vi "CHeckHardware.vi"(3 "Hardware":path) -> (1 "HardwareSpecs":T1)   [LabVIEW 2012]
uses:
  <userlib>/BotSpeak/VIs/SubVIs/BotSpeak.HardwareSpecs.ctl
  <userlib>/BotSpeak/VIs/SubVIs/BotSpeak_Globals.vi
panel:
  out "path":path
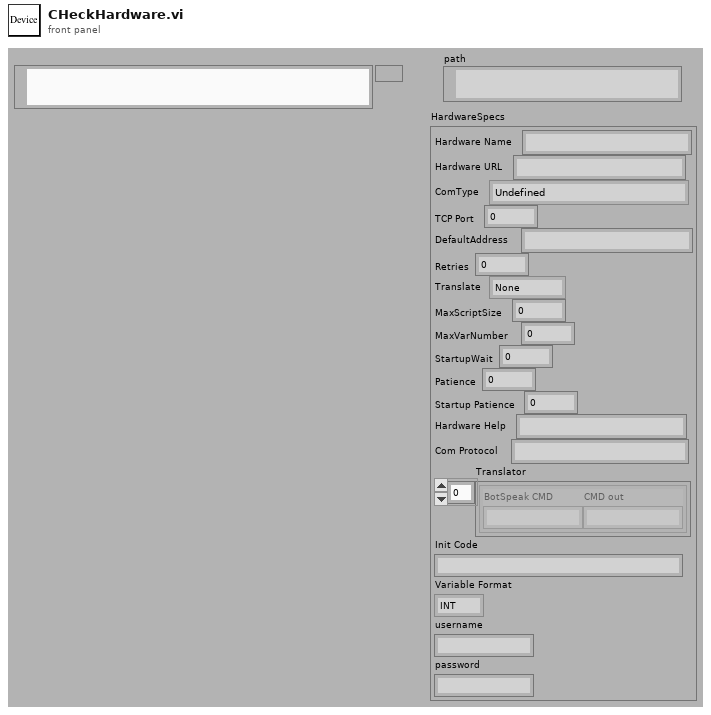
[diagram p1: front panel]
types:
  T1 = typedef "BotSpeak.HardwareSpecs.ctl" = cluster{"Hardware Name":string, "Hardware URL":string, "ComType":enum16{"Undefined", "Serial", "TCPIP", "Console", "EV3"}, "TCP Port":i32, "DefaultAddress":string, "Retries":i32, "Translate":enum16{"None", "Tiny", "URAPI"}, "MaxScriptSize":i32, "MaxVarNumber":i32, "StartupWait":i32, "Patience":i32, "Startup Patience":i32, "Hardware Help":string, "Com Protocol":string, "Translator":cluster{"BotSpeak CMD":string, "CMD out":string}[], "Init Code":string, "Variable Format":enum16{"INT", "FLOAT", "FIXED"}, "username":string, "password":string}
  T2 = typedef "BotSpeak_Control.ctl" = cluster{"Address":string, "Reply EOF":string, "Hardware":string, "Retries":i8, "Timeout":i32, "Open?":bool}
  T3 = cluster{"trimmed string":string, "trimmed string":string}[]
  T4 = cluster{"trimmed string":string, "trimmed string":string}
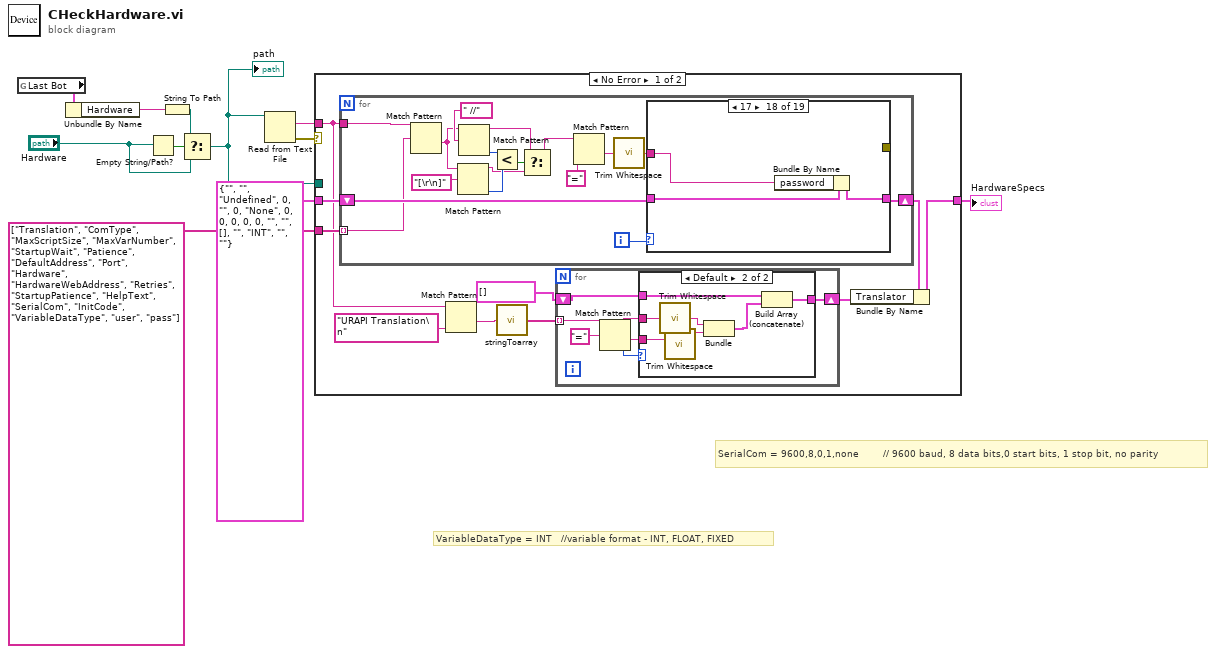
[diagram p0: block diagram]
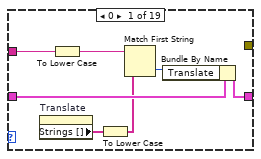
[diagram p3: hidden frame]
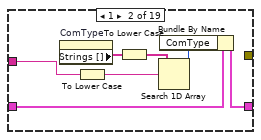
[diagram p4: hidden frame]
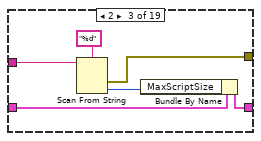
[diagram p5: hidden frame]
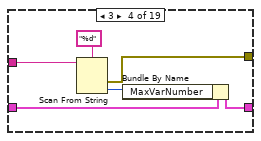
[diagram p6: hidden frame]
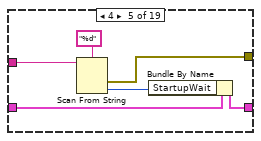
[diagram p7: hidden frame]
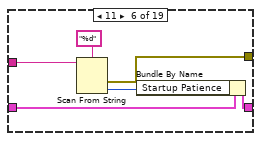
[diagram p8: hidden frame]
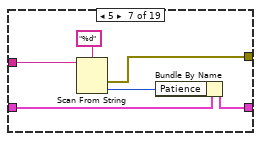
[diagram p9: hidden frame]
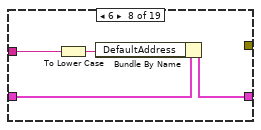
[diagram p10: hidden frame]
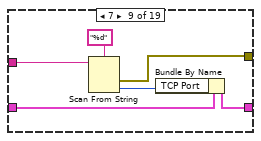
[diagram p11: hidden frame]
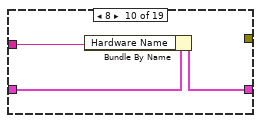
[diagram p12: hidden frame]
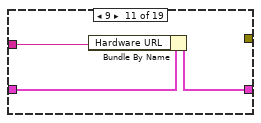
[diagram p13: hidden frame]
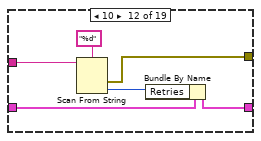
[diagram p14: hidden frame]
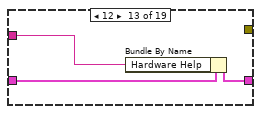
[diagram p15: hidden frame]
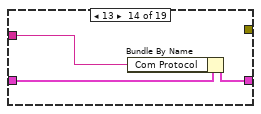
[diagram p16: hidden frame]
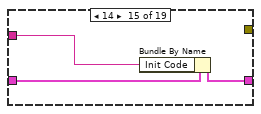
[diagram p17: hidden frame]
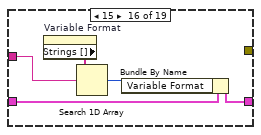
[diagram p18: hidden frame]
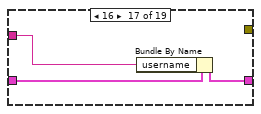
[diagram p19: hidden frame]
diagram:
  # "VariableDataType = INT   //variable format - INT, FLOAT, FIXED"
  # "SerialCom = 9600,8,0,1,none        // 9600 baud, 8 data bits,0 start bits, 1 stop bit, no parity"
  n1 = global read "BotSpeak_Globals.vi" "Last Bot"() -> (w6:T2)
  n2 = Unbundle By Name(w6) -> ("Hardware"=w2:string)
  n3 = Empty String/Path?(string/path="Hardware") -> (empty?=w5:bool)
  n4 = String To Path(string=w2) -> (path=w1:path)
  n5 = Select(t=w1, s=w5, f="Hardware") -> (s? t:f=w3:path)
  "path" <- w3
  n6 = Read from Text File(file (use dialog)=w3) -> (text=w10:string, error out=w11:errorcluster)  [unwired: 3 in, 2 out]
  n7 = case shown="No Error" w11 {
    tunnel: w3 -> [_ w142]
    tunnel: string[] ["Translation", "ComType", "MaxScriptSize", "MaxVarNumber", "StartupWait", "Patience", "DefaultAddress", "Port", "Hardware", "HardwareWebAddress", "Retries", "StartupPatience", "HelpText", "SerialCom", "InitCode", "VariableDataType", "user", "pass"] -> [w21 _]
    tunnel: w10 -> [w19 _]
    tunnel: T1 {"Hardware Name"="", "Hardware URL"="", "ComType"=enum."Undefined", "TCP Port"=0, "DefaultAddress"="", "Retries"=0, "Translate"=enum."None", "MaxScriptSize"=0, "MaxVarNumber"=0, "StartupWait"=0, "Patience"=0, "Startup Patience"=0, "Hardware Help"="", "Com Protocol"="", "Translator"=[], "Init Code"="", "Variable Format"=enum."INT", "username"="", "password"=""} ("HardwareSpecs") -> [w20 w141]
    tunnel: [w14 w141] -> w8
    frame No Error {
      n8 = for {
        tunnel: w21 -> [w42] mode=indexing
        tunnel: w19 -> [w41]
        shift-right: [w49] -> w15
        shift-left: w20 -> [w50]
        i -> [w51]
        n9 = Match Pattern(string=w41, regular expression=w42) -> (after substring=w45:string)  [unwired: 1 in, 3 out]
        n10 = Match Pattern(string=w45, regular expression="[\r\n]") -> (before substring=w39:string, offset past match=w43:i32)  [unwired: 1 in, 2 out]
        n11 = Match Pattern(string=w45, regular expression=" //") -> (before substring=w40:string, offset past match=w44:i32)  [unwired: 1 in, 2 out]
        n12 = Less?(x=w44, y=w43) -> (x < y?=w38:bool)
        n13 = Select(t=w40, s=w38, f=w39) -> (s? t:f=w37:string)
        n14 = Match Pattern(string=w37, regular expression="=") -> (after substring=w52:string)  [unwired: 1 in, 3 out]
        n15 = call <vilib>:"Trim Whitespace.vi"("string"=w52) -> ("trimmed string"=w48:string)  [unwired: 1 in]
        n16 = case shown="17" w51 {
          tunnel: w50 -> [w60 w67 w73 w79 w85 w91 w97 w101 w107 w110 w113 w119 w122 w125 w128 w133 w136 w139 w140]
          tunnel: [w59 w66 w72 w78 w84 w90 w96 w100 w106 w109 w112 w118 w121 w124 w127 w132 w135 w138 w140] -> w49
          tunnel: w48 -> [w58 w65 w71 w77 w83 w89 w95 w99 w105 w108 w111 w117 w120 w123 w126 w130 w134 w137 _]
          tunnel: [_ _ w68 w74 w80 w86 w92 _ w102 _ _ w114 _ _ _ _ _ _ _] -> _
          frame 0 {
            n17 = property on="Translate" class="Enum (strict)"() -> ("Strings []"=w56:string[])  [unwired: 2 in, 2 out]
            n18 = To Lower Case(string=w58) -> (all lower case string=w57:string)
            n19 = To Lower Case(string=w56) -> (all lower case string=w54:string[])
            n20 = Match First String(2:w54, 3:w57) -> (0:w55:i32)  [unwired: 1 out]
            n21 = Bundle By Name(cluster=w60, "Translate"=w55) -> (w59:T1)
          }
          frame 1 {
            n22 = property on="ComType" class="Enum (strict)"() -> ("Strings []"=w62:string[])  [unwired: 2 in, 2 out]
            n23 = To Lower Case(string=w65) -> (all lower case string=w61:string)
            n24 = To Lower Case(string=w62) -> (all lower case string=w63:string[])
            n25 = Search 1D Array(1D array=w63, element=w61) -> (index of element=w64:i32)  [unwired: 1 in]
            n26 = Bundle By Name(cluster=w67, "ComType"=w64) -> (w66:T1)
          }
          frame 2 {
            n27 = Scan From String(format string="%d", input string=w71) -> (error out=w68:errorcluster, output 1=w70:i32)  [unwired: 3 in, 2 out]
            n28 = Bundle By Name(cluster=w73, "MaxScriptSize"=w70) -> (w72:T1)
          }
          frame 3 {
            n29 = Scan From String(format string="%d", input string=w77) -> (error out=w74:errorcluster, output 1=w76:i32)  [unwired: 3 in, 2 out]
            n30 = Bundle By Name(cluster=w79, "MaxVarNumber"=w76) -> (w78:T1)
          }
          frame 4 {
            n31 = Scan From String(format string="%d", input string=w83) -> (error out=w80:errorcluster, output 1=w82:i32)  [unwired: 3 in, 2 out]
            n32 = Bundle By Name(cluster=w85, "StartupWait"=w82) -> (w84:T1)
          }
          frame 11 {
            n33 = Scan From String(format string="%d", input string=w89) -> (error out=w86:errorcluster, output 1=w88:i32)  [unwired: 3 in, 2 out]
            n34 = Bundle By Name(cluster=w91, "Startup Patience"=w88) -> (w90:T1)
          }
          frame 5 {
            n35 = Scan From String(format string="%d", input string=w95) -> (error out=w92:errorcluster, output 1=w94:i32)  [unwired: 3 in, 2 out]
            n36 = Bundle By Name(cluster=w97, "Patience"=w94) -> (w96:T1)
          }
          frame 6 {
            n37 = To Lower Case(string=w99) -> (all lower case string=w98:string)
            n38 = Bundle By Name(cluster=w101, "DefaultAddress"=w98) -> (w100:T1)
          }
          frame 7 {
            n39 = Scan From String(format string="%d", input string=w105) -> (error out=w102:errorcluster, output 1=w103:i32)  [unwired: 3 in, 2 out]
            n40 = Bundle By Name(cluster=w107, "TCP Port"=w103) -> (w106:T1)
          }
          frame 8 {
            n41 = Bundle By Name(cluster=w110, "Hardware Name"=w108) -> (w109:T1)
          }
          frame 9 {
            n42 = Bundle By Name(cluster=w113, "Hardware URL"=w111) -> (w112:T1)
          }
          frame 10 {
            n43 = Scan From String(format string="%d", input string=w117) -> (error out=w114:errorcluster, output 1=w116:i32)  [unwired: 3 in, 2 out]
            n44 = Bundle By Name(cluster=w119, "Retries"=w116) -> (w118:T1)
          }
          frame 12 {
            n45 = Bundle By Name(cluster=w122, "Hardware Help"=w120) -> (w121:T1)
          }
          frame 13 {
            n46 = Bundle By Name(cluster=w125, "Com Protocol"=w123) -> (w124:T1)
          }
          frame 14 {
            n47 = Bundle By Name(cluster=w128, "Init Code"=w126) -> (w127:T1)
          }
          frame 15 {
            n48 = property on="Variable Format" class="Enum (strict)"() -> ("Strings []"=w131:string[])  [unwired: 2 in, 2 out]
            n49 = Search 1D Array(1D array=w131, element=w130) -> (index of element=w129:i32)  [unwired: 1 in]
            n50 = Bundle By Name(cluster=w133, "Variable Format"=w129) -> (w132:T1)
          }
          frame 16 {
            n51 = Bundle By Name(cluster=w136, "username"=w134) -> (w135:T1)
          }
          frame 17 {
            n52 = Bundle By Name(cluster=w139, "password"=w137) -> (w138:T1)
          }
          frame Default {
          }
        }
      }
      n53 = Match Pattern(string=w19, regular expression="URAPI Translation\n") -> (after substring=w17:string)  [unwired: 1 in, 3 out]
      n54 = call <userlib>:"stringToarray.vi"("String"=w17) -> ("Array"=w16:string[])
      n55 = for {
        tunnel: w16 -> [w27] mode=indexing
        shift-right: [w23] -> w12
        shift-left: T3 [] -> [w22]
        n56 = Match Pattern(string=w27, regular expression="=") -> (before substring=w26:string, after substring=w25:string, offset past match=w24:i32)  [unwired: 1 in, 1 out]
        n57 = case shown="Default" w24 {
          tunnel: w26 -> [_ w36]
          tunnel: w25 -> [_ w35]
          tunnel: [w29 w31] -> w23
          tunnel: w22 -> [w29 w30]
          frame -1 {
          }
          frame Default {
            n58 = call <vilib>:"Trim Whitespace.vi"("string"=w36) -> ("trimmed string"=w34:string)  [unwired: 1 in]
            n59 = call <vilib>:"Trim Whitespace.vi"("string"=w35) -> ("trimmed string"=w33:string)  [unwired: 1 in]
            n60 = Bundle("trimmed string"=w34, "trimmed string"=w33) -> (w32:T4)  [unwired: 1 in]
            n61 = Build Array (concatenate)(w30, w32) -> (w31:T3)
          }
        }
      }
      n62 = Bundle By Name(cluster=w15, "Translator"=w12) -> (w14:T1)
    }
    frame Error {
      n63 = disable-structure shown="Disabled" {
        disable-tunnel: w142 -> [w145 _]
        frame Disabled {
          n64 = Format Into String(format string="No such hardware: %s", w145) -> (resulting string=w144:string)  [unwired: 2 in, 1 out]
          n65 = One Button Dialog(message=w144) -> ()  [unwired: 1 in, 1 out]
        }
        frame Enabled {
        }
      }
    }
  }
  "HardwareSpecs" <- w8
